vi "Increment Clones.vi"(8 "error in (no error)":errorcluster, 11 "Service in":refnum<class "Service.lvclass">) -> (0 "error out":errorcluster, 3 "Service out":refnum<class "Service.lvclass">)   [LabVIEW 2024, in "Ramses Framework.lvlib" / "Service.lvclass"]
uses:
  Service.lvclass
  Service.lvclass/Service.ctl
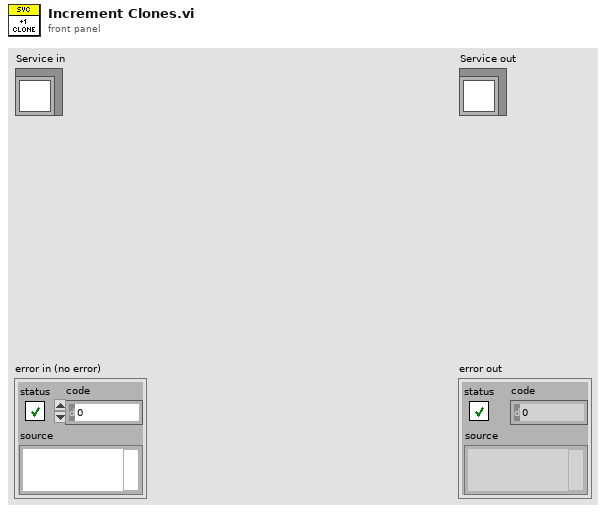
[diagram p1: front panel]
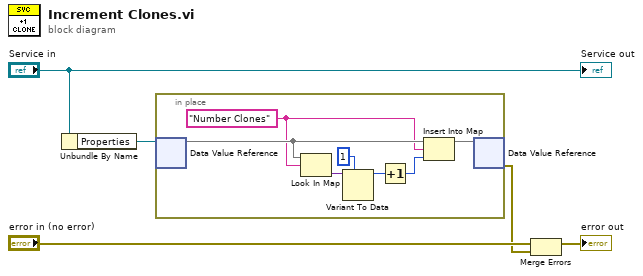
[diagram p0: block diagram]
diagram:
  n1 = Unbundle By Name("Service in") -> ("Properties"=w4:refnum<data-value>)
  n2 = in-place {
    w8 = "Number Clones" ("Key")
    n3 = in-place-dvr #1(w4) -> (w9:map{string, variant})  [unwired: 1 out]
    n4 = Look In Map(map=w9, key=w8) -> (value=w12:variant)  [unwired: 1 in, 1 out]
    n5 = Variant To Data(type=1, Variant=w12) -> (data=w10:i32)  [unwired: 1 in, 1 out]
    n6 = Increment(x=w10) -> (x+1=w7:i32)
    n7 = Insert Into Map(map in=w9, key=w8, value=w7) -> (map out=w6:map{string, variant})  [unwired: 2 out]
    n8 = in-place-dvr #1(w6) -> (w1:errorcluster)  [unwired: 1 out]
  }
  n9 = Merge Errors("error in (no error)", w1) -> (→"error out":errorcluster)
  "Service out" <- "Service in"
